vi "配置控件.vi"(8 "error in (no error)":errorcluster caption="错误输入（无错误）", 11 "程序 输入":refnum<class "程序.lvclass">) -> (0 "error out":errorcluster caption="错误输出", 3 "程序 输出":refnum<class "程序.lvclass">)   [LabVIEW 2018, in "程序.lvclass"]
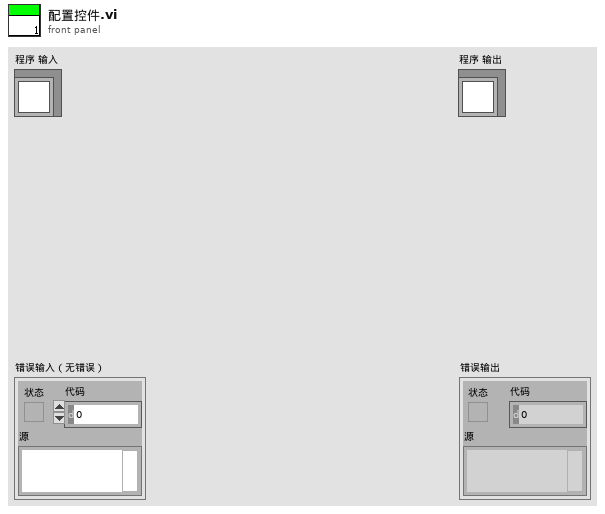
[diagram p1: front panel]
types:
  T1 = typedef "LVPoint32TypeDef.ctl" = cluster{"Horizontal":i32, "Vertical":i32}
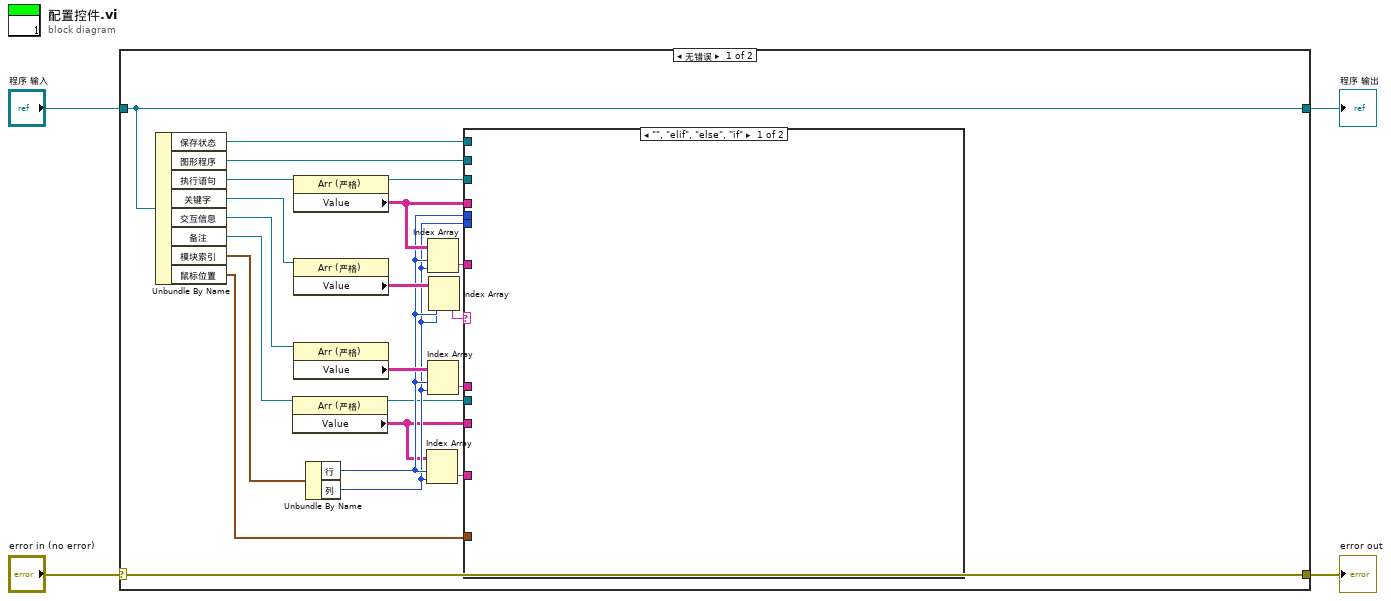
[diagram p0: block diagram]
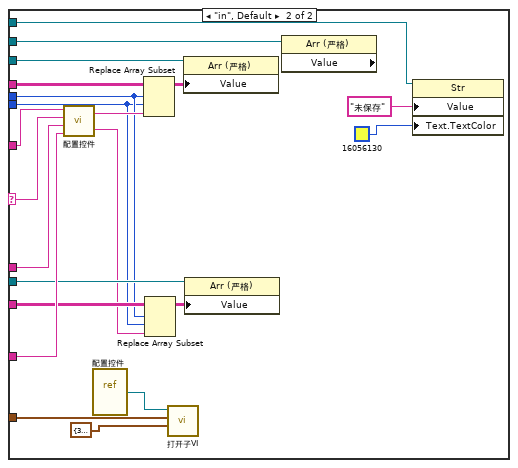
[diagram p2: hidden frame]
diagram:
  n1 = case shown="无错误" "error in (no error)" {
    selector: "error in (no error)" -> [w26 w49]
    tunnel: [w26 w49] -> w3
    tunnel: [w25 w48] -> w1
    tunnel: "程序 输入" -> [w25 w48]
    frame No Error {
      n2 = Unbundle By Name(w25) -> ("保存状态"=w5:refnum<vi>, "图形程序"=w6:refnum<vi>, "执行语句"=w21:refnum<vi>, "关键字"=w15:refnum<vi>, "交互信息"=w24:refnum<vi>, "备注"=w13:refnum<vi>, "模块索引"=w22:cluster{"列":u32, "行":u32}, "鼠标位置"=w17:T1)
      n3 = property class="Arr (严格)"(reference=w13) -> (reference out=w7:refnum<vi>, "Value"=w8:string[][])  [unwired: 1 in, 1 out]
      n4 = property class="Arr (严格)"(reference=w21) -> (reference out=w19:refnum<vi>, "Value"=w18:string[][])  [unwired: 1 in, 1 out]
      n5 = property class="Arr (严格)"(reference=w15) -> ("Value"=w16:string[][])  [unwired: 1 in, 2 out]
      n6 = property class="Arr (严格)"(reference=w24) -> ("Value"=w23:string[][])  [unwired: 1 in, 2 out]
      n7 = Unbundle By Name(w22) -> ("行"=w12:u32, "列"=w11:u32)
      n8 = Index Array(array=w8, index (row)=w12, index (col)=w11) -> (element=w10:string)
      n9 = Index Array(array=w18, index (row)=w12, index (col)=w11) -> (element=w20:string)
      n10 = Index Array(array=w23, index (row)=w12, index (col)=w11) -> (element=w14:string)
      n11 = Index Array(array=w16, index (row)=w12, index (col)=w11) -> (element=w9:string)
      n12 = case shown="\"\", \"elif\", \"else\", \"if\"" w9 {
        selector: w9 -> [_ w39]
        tunnel: w20 -> [_ w47]
        tunnel: w14 -> [_ w38]
        tunnel: w19 -> [_ w46]
        tunnel: w18 -> [_ w45]
        tunnel: w17 -> [_ w41]
        tunnel: w12 -> [_ w32]
        tunnel: w11 -> [_ w31]
        tunnel: w10 -> [_ w40]
        tunnel: w8 -> [_ w36]
        tunnel: w7 -> [_ w35]
        tunnel: w6 -> [_ w33]
        tunnel: w5 -> [_ w29]
        frame "", "elif", "else", "if" {
        }
        frame "in", Default {
          n13 = call "配置控件.vi"("原备注"=w40, "交互信息"=w38, "关键字"=w39, "原值"=w47) -> ("新备注"=w30:string, "新值"=w37:string)  [unwired: 2 in]
          n14 = vi-ref "配置控件.vi"() -> (w43:refnum<vi>)
          n15 = Replace Array Subset(array=w45, new element=w37, index (row)=w32, index (col)=w31) -> (w44:string[][])
          n16 = Replace Array Subset(array=w36, new element=w30, index (row)=w32, index (col)=w31) -> (w34:string[][])
          n17 = call "打开子VI.vi"("窗口大小"=cluster{"wide":i32, "Top":i32} {"wide"=313, "Top"=143}, "窗口位置"=w41, "引用"=w43) -> ()  [unwired: 7 in, 2 out]
          n18 = property class="Arr (严格)"(reference=w46, "Value"=w44) -> ()  [unwired: 1 in, 2 out]
          n19 = property class="Arr (严格)"(reference=w35, "Value"=w34) -> ()  [unwired: 1 in, 2 out]
          n20 = property class="Arr (严格)" props=["Value"](reference=w33) -> ()  [unwired: 1 in, 3 out]
          n21 = property class="Str"(reference=w29, "Value"="未保存" ("值"), "Text.TextColor"=u32 16056130) -> ()  [unwired: 1 in, 2 out]
        }
      }
    }
    frame Error {
    }
  }
  "error out" <- w3
  "程序 输出" <- w1
